vi "get_POSs.vi"(8 "error in (no error)":errorcluster caption="错误输入（无错误）", 11 "MotorSystem 输入":refnum<class "MotorSystem.lvclass">) -> (0 "error out":errorcluster caption="错误输出", 2 "pos":dbl[](array[numeric]), 3 "MotorSystem 输出":refnum<class "MotorSystem.lvclass">)   [LabVIEW 2016, in "MotionControl_UFO_3DOF.lvlib" / "MotorSystem.lvclass"]
uses:
  <userlib>/MotionControl_UFO_3DOF/MotorSystem/MotorSystem.lvclass
  <userlib>/MotionControl_UFO_3DOF/MotorSystem/MotorSystem.lvclass/MotorSystem.ctl
  <userlib>/MotionControl_UFO_3DOF/OneMotion/OneMotion.lvclass
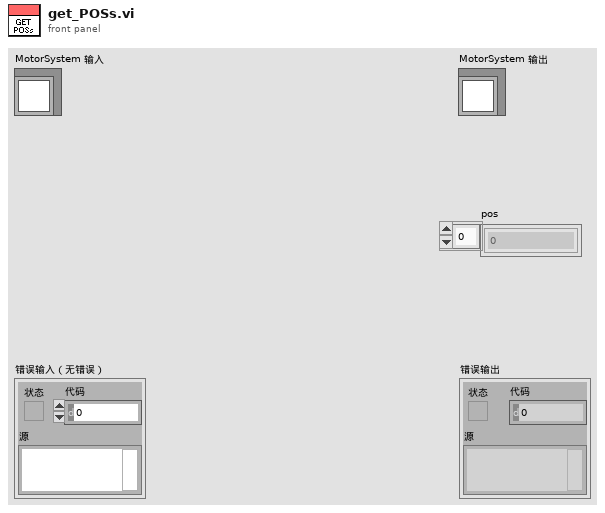
[diagram p1: front panel]
types:
  T1 = typedef "MotionControl_UFO_3DOF.lvlib/MotorSystem.lvclass/MotionCluster.ctl" = cluster{"OneMotion.lvclass":refnum<class "OneMotion.lvclass">, "connected?":bool, "default enabled?":bool, "enabled?":bool}
  T2 = typedef "MotionControl_UFO_3DOF.lvlib/OneMotion.lvclass/unit mode.ctl" = enum16{"motor (pulse)", "linear (mm) or radial (degree)"}
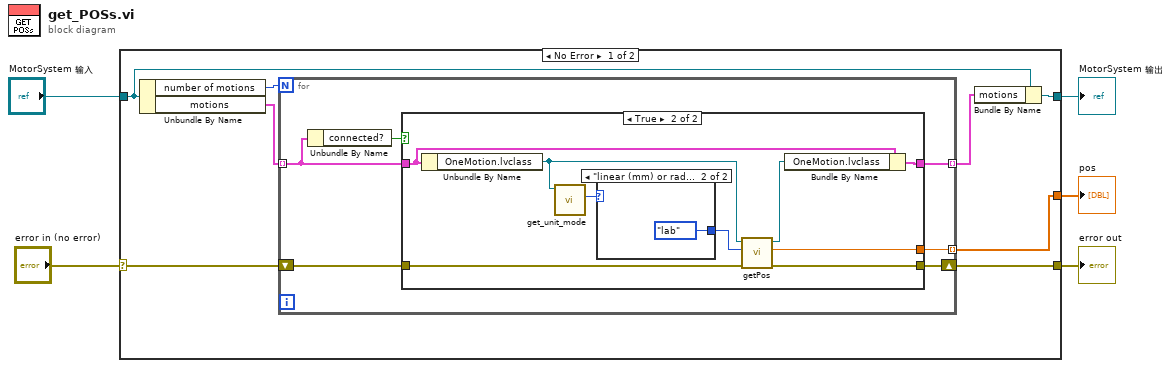
[diagram p0: block diagram]
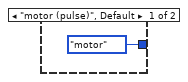
[diagram p3: hidden frame]
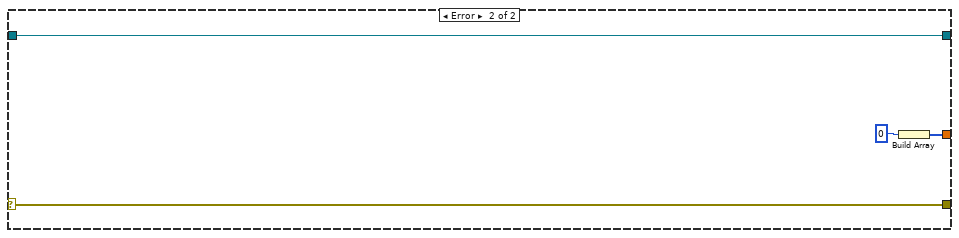
[diagram p4: hidden frame]
diagram:
  n1 = case shown="No Error" "error in (no error)" {
    selector: "error in (no error)" -> [w11 w36]
    tunnel: [w10 w36] -> w4
    tunnel: [w7 w35] -> w2
    tunnel: "MotorSystem 输入" -> [w9 w35]
    tunnel: [w12 w33] -> w1
    frame No Error {
      n2 = Unbundle By Name(w9) -> ("number of motions"=w13:i32, "motions"=w6:T1[])
      n3 = for {
        N: w13 -> [_]
        tunnel: w6 -> [w15] mode=indexing
        tunnel: [w17] -> w12 mode=indexing
        shift-right: [w18] -> w10
        shift-left: w11 -> [w19]
        tunnel: [w16] -> w8 mode=indexing
        n4 = Unbundle By Name(w15) -> ("connected?"=w14:bool)
        n5 = case shown="True" w14 {
          tunnel: w19 -> [w20 w30]
          tunnel: [w20 w29] -> w18
          tunnel: [_ w28] -> w17
          tunnel: [w21 w26] -> w16
          tunnel: w15 -> [w21 w22]
          frame False {
          }
          frame True {
            n6 = Unbundle By Name(w22) -> ("OneMotion.lvclass"=w25:refnum<class "OneMotion.lvclass">)
            n7 = call-dynamic "get_unit_mode.vi"("OneMotion输入"=w25) -> ("unit mode"=w24:T2)  [unwired: 8 in, 2 out]
            n8 = case shown="\"linear (mm) or radial (degree)\"" w24 {
              tunnel: [enum16{"lab", "motor"}."motor" ("lab or motor") enum16{"lab", "motor"}."lab" ("lab or motor")] -> w23
              frame "motor (pulse)", Default {
              }
              frame "linear (mm) or radial (degree)" {
              }
            }
            n9 = call <userlib>:"getPos.vi"("error in (no error)"=w30, "lab or motor"=w23, "OneMotion 输入"=w25) -> ("error out"=w29:errorcluster, "pos"=w28:dbl, "OneMotion 输出"=w27:refnum<class "OneMotion.lvclass">)  [unwired: 6 in]
            n10 = Bundle By Name(cluster=w22, "OneMotion.lvclass"=w27) -> (w26:T1)
          }
        }
      }
      n11 = Bundle By Name(cluster=w9, "motions"=w8) -> (w7:refnum<class "MotorSystem.lvclass">)
    }
    frame Error {
      n12 = Build Array(0) -> (w33:i32[])
    }
  }
  "error out" <- w4
  "MotorSystem 输出" <- w2
  "pos" <- w1
